vi "PC_Main.vi"() -> ()   [LabVIEW 2018]
uses:
  Type Defs/measurement states.ctl
  Type Defs/Processing Settings 1.ctl
  <vilib>/Analysis/baseanly.llb/Mean (DBL).vi
  <vilib>/WebDAVClient/Simple Get Buffer.vi
  <vilib>/WebDAVClient/NI_WebDAV.lvlib
  Alignment Mode Window.vi
  Update Settings.vi
  <vilib>/Analysis/NI_AALBase.lvlib
panel:
  in  "Settings":bool
  in  "Alignment":bool
  in  "Start Button":bool
  in  "STOP":bool
  in  "Choose Correction":bool caption="Calculated              Calibration\nCorrection                Correction"
  in  "Sensor Select":bool
  in  "Repeat\nMeasurement":bool
  out "Meas. Complete":bool
  out "Waiting For Data":bool
  out "Detection Failure":bool=TRUE
  out "Peaks":cluster{"Locations":dbl[], "Amplitudes":dbl[]}[](graph)
  out "Mean Thickness (µm)":dbl format="%.2g"
  out "Thickness Array":dbl[](array[numeric]) format="%.2g"
  in  "N Tests":i32
  in  "alignment off":bool
  out "Thickness (µm)":dbl format="%.2g"
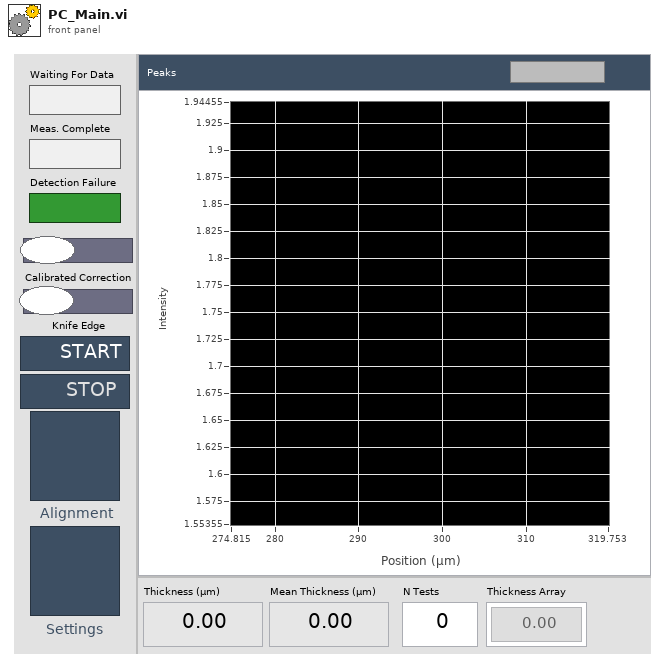
[diagram p1: front panel]
types:
  T1 = typedef "Processing Settings 1.ctl" = cluster{"Edlen\nSettings":cluster{"P_atm":i32, "T (deg C)":i32, "PP h20":dbl}, "Processing\nSettings":cluster{"Subset Length":i32, "Peak Width":i32, "Filter Width":i32, "Threshold (V)":dbl}}
  T2 = typedef "measurement states.ctl" = enum16{"reset alignment mode", "sensor select", "start measurement", "alignment", "configure", "idle", "wait for data", "load data", "process data", "exit", "find peaks"}
  T3 = cluster{"Moving Averaged Array":dbl[], "Moving Averaged Array":dbl[]}
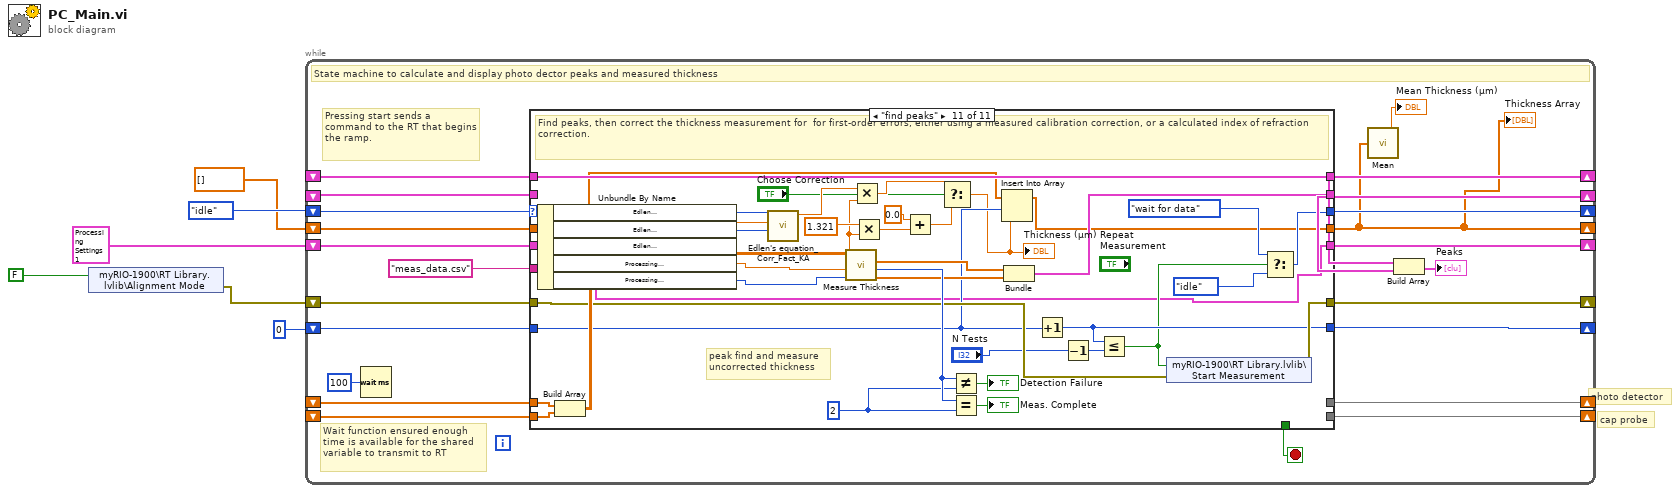
[diagram p0: block diagram]
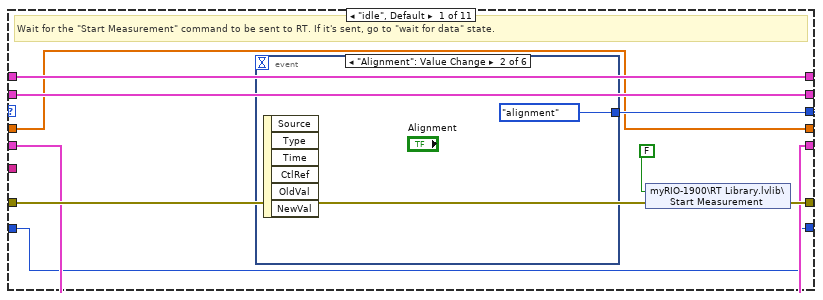
[diagram p2: hidden frame]
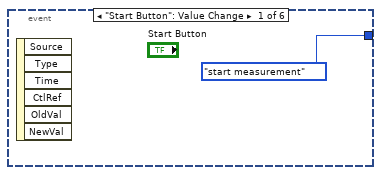
[diagram p3: hidden frame]
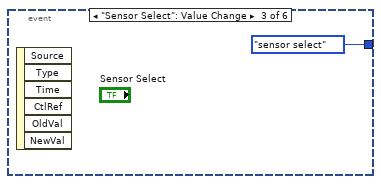
[diagram p4: hidden frame]
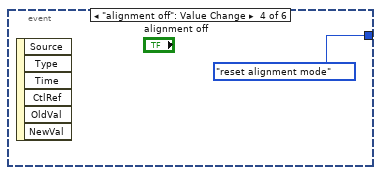
[diagram p5: hidden frame]
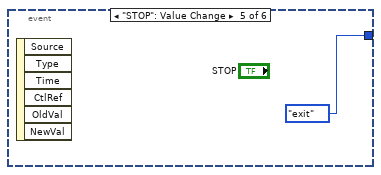
[diagram p6: hidden frame]
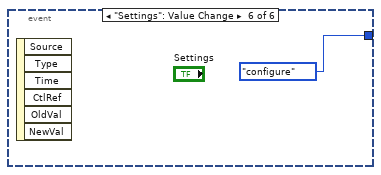
[diagram p7: hidden frame]
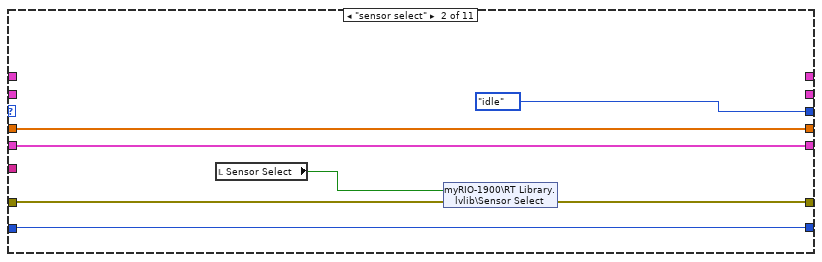
[diagram p8: hidden frame]
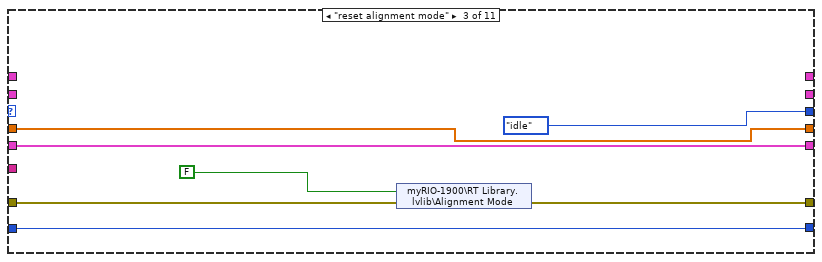
[diagram p9: hidden frame]
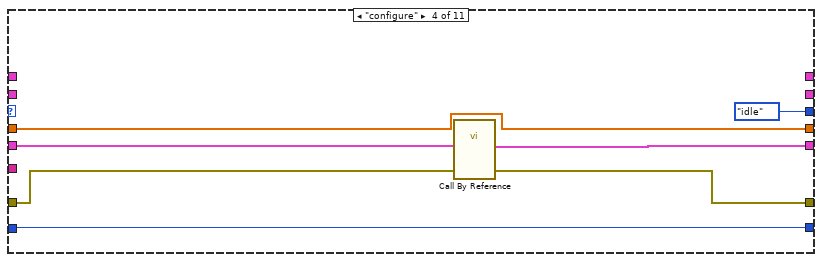
[diagram p10: hidden frame]
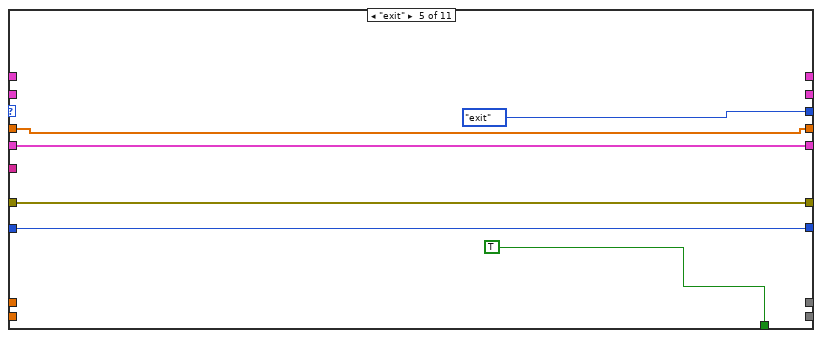
[diagram p11: hidden frame]
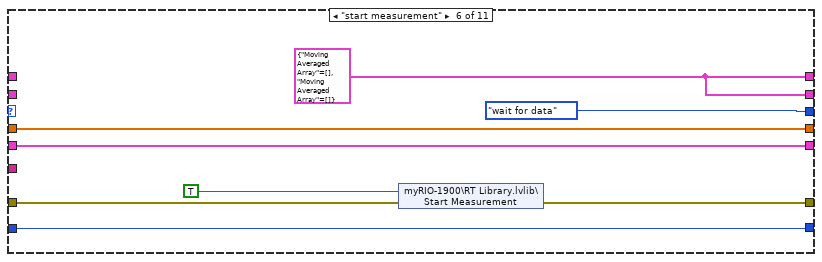
[diagram p12: hidden frame]
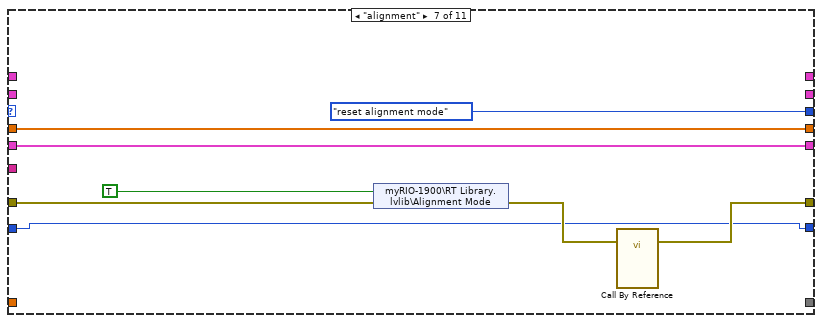
[diagram p13: hidden frame]
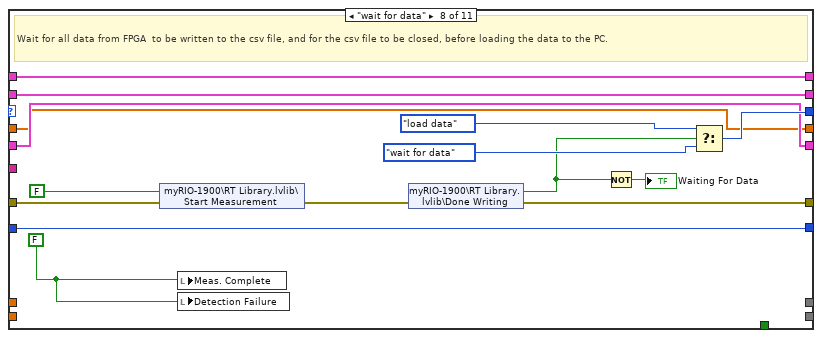
[diagram p14: hidden frame]
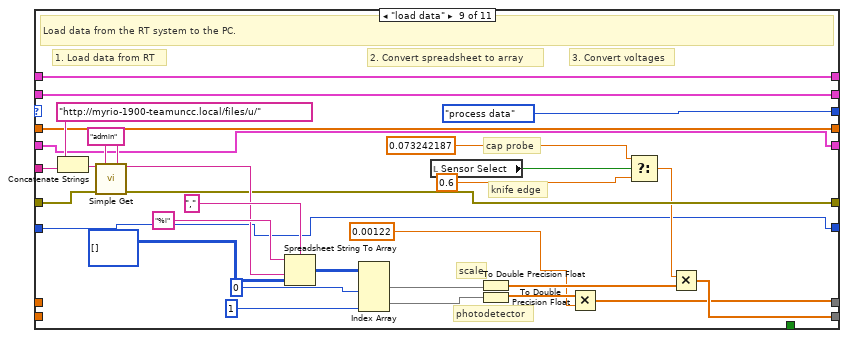
[diagram p15: hidden frame]
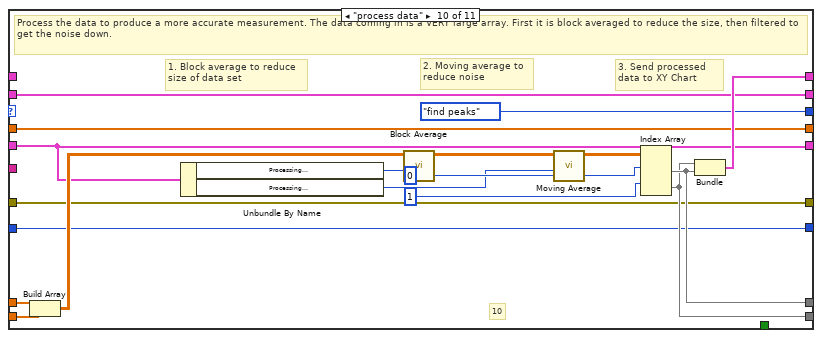
[diagram p16: hidden frame]
diagram:
  # "photo detector"
  # "cap probe"
  n1 = shared-variable "myRIO-1900\\RT Library.lvlib\\Alignment Mode"(FALSE) -> (error out=w4:errorcluster)  [unwired: 1 in]
  n2 = while {
    shift-right: [w28] -> _
    shift-left: measurement_states."idle" ("Enum") -> [w29]
    shift-right: [w27] -> _
    shift-left: w4 -> [w15]
    shift-right: [w25] -> _
    shift-left: _ -> [w24]
    shift-right: [w26] -> _
    shift-left: _ -> [w23]
    shift-right: [w18] -> _
    shift-left: _ -> [w17]
    shift-right: [w19] -> _
    shift-left: _ -> [w16]
    shift-right: [w10] -> _
    shift-left: dbl[] [] -> [w13]
    shift-right: [w11] -> _
    shift-left: 0 -> [w12]
    shift-right: [w7] -> _
    shift-left: T1 {"Edlen\nSettings"={"P_atm"=100, "T (deg C)"=50, "PP h20"=100.0}, "Processing\nSettings"={"Subset Length"=1, "Peak Width"=50, "Filter Width"=100, "Threshold (V)"=0.8}} ("Processing\nSettings") -> [w8]
    stop <- w14 stop-if-true
    # "Wait function ensured enough time is available for the shared variable to transmit to RT"
    # "Pressing start sends a command to the RT that begins the ramp."
    # "State machine to calculate and display photo dector peaks and measured thickness"
    n3 = Wait (ms)(milliseconds to wait=u32 100) -> ()  [unwired: 1 out]
    n4 = case shown="\"find peaks\"" w29 {
      tunnel: [w36 measurement_states."idle" ("Enum") measurement_states."idle" ("Enum") measurement_states."idle" ("Enum") measurement_states."exit" ("Enum") measurement_states."wait for data" ("Enum") measurement_states."reset alignment mode" ("Enum") w101 measurement_states."process data" measurement_states."find peaks" w175] -> w28
      tunnel: [w33 w50 w56 w63 w68 w79 w83 w97 w120 w141 w173] -> w27
      tunnel: [_ _ _ _ _ _ _ _ w117 w142 _] -> w25
      tunnel: [_ _ _ _ _ _ _ _ w114 w143 _] -> w26
      tunnel: w24 -> [_ _ _ _ _ _ _ _ _ w148 w187]
      tunnel: w23 -> [_ _ _ _ _ _ _ _ _ w149 w188]
      tunnel: "meas_data.csv" ("File Name") -> [_ _ _ _ _ _ _ _ w118 _ _]
      tunnel: w15 -> [w34 w51 w57 w64 w68 w78 w87 w92 w113 w141 w174]
      tunnel: [w38 _ _ _ _ w74 _ w94 w112 w140 w178] -> w19
      tunnel: [w37 _ _ _ _ w74 _ w95 w111 w139 w179] -> w18
      tunnel: w17 -> [w37 _ _ _ _ _ _ w95 w111 w139 _]
      tunnel: w16 -> [w38 _ _ _ _ _ _ w94 w112 _ w178]
      tunnel: [_ _ _ _ TRUE _ _ _ _ _ _] -> w14
      tunnel: w8 -> [w32 w47 w54 w59 w69 w75 w82 w90 w106 w135 w158]
      tunnel: [w32 w47 w54 w60 w69 w75 w82 w90 w106 w135 w158] -> w7
      tunnel: [w31 w46 w53 w62 w67 w73 w81 w89 w105 w134 w172] -> w10
      tunnel: w13 -> [w31 w46 w53 w62 w67 w73 w81 w89 w105 w134 w171]
      tunnel: w12 -> [w30 w45 w52 w61 w66 w72 w80 w88 w104 w133 w170]
      tunnel: [w30 w45 w52 w61 w66 w72 w80 w88 w104 w133 w169] -> w11
      frame "idle", Default {
        # "Wait for the \"Start Measurement\" command to be sent to RT. If it's sent, go to \"wait for data\" state."
        n5 = event shown="[1] \"Alignment\": Value Change" {
          selector: _ -> [_ _ _ _ _ _]
          dyn-events: _ -> [_ _ _ _ _ _]
          timeout: _ -> [_ _ _ _ _ _]
          tunnel: [measurement_states."start measurement" ("Enum") measurement_states."alignment" ("Enum") measurement_states."sensor select" ("Enum") measurement_states."reset alignment mode" ("Enum") measurement_states."exit" ("Enum") measurement_states."configure" ("Enum")] -> w36
          event "Start Button": Value Change {
            n6 = event-data() -> ()  [unwired: 1 in, 6 out]
          }
          event "Alignment": Value Change {
            n7 = event-data() -> ()  [unwired: 1 in, 6 out]
          }
          event "Sensor Select": Value Change {
            n8 = event-data() -> ()  [unwired: 1 in, 6 out]
          }
          event "alignment off": Value Change {
            n9 = event-data() -> ()  [unwired: 1 in, 6 out]
          }
          event "STOP": Value Change {
            n10 = event-data() -> ()  [unwired: 1 in, 6 out]
          }
          event "Settings": Value Change {
            n11 = event-data() -> ()  [unwired: 1 in, 6 out]
          }
        }
        n12 = shared-variable "myRIO-1900\\RT Library.lvlib\\Start Measurement"(FALSE, error in=w34) -> (error out=w33:errorcluster)
      }
      frame "sensor select" {
        n13 = local read "Sensor Select"() -> (w49:bool)
        n14 = shared-variable "myRIO-1900\\RT Library.lvlib\\Sensor Select"(w49, error in=w51) -> (error out=w50:errorcluster)
      }
      frame "reset alignment mode" {
        n15 = shared-variable "myRIO-1900\\RT Library.lvlib\\Alignment Mode"(FALSE, error in=w57) -> (error out=w56:errorcluster)
      }
      frame "configure" {
        n16 = call-by-ref "?"("error in (no error)"=w64, "Processing\nSettings 2"=w59) -> ("error out"=w63:errorcluster, "Processing\nSettings Out"=w60:T1)  [unwired: 10 in, 2 out]
      }
      frame "exit" {
      }
      frame "start measurement" {
        w74 = T3 {"Moving Averaged Array"=[], "Moving Averaged Array"=[]}
        n17 = shared-variable "myRIO-1900\\RT Library.lvlib\\Start Measurement"(TRUE, error in=w78) -> (error out=w79:errorcluster)
      }
      frame "alignment" {
        n18 = shared-variable "myRIO-1900\\RT Library.lvlib\\Alignment Mode"(TRUE, error in=w87) -> (error out=w84:errorcluster)
        n19 = call-by-ref "?"(error in=w84) -> (error out=w83:errorcluster)  [unwired: 13 in, 1 out]
      }
      frame "wait for data" {
        w96 = FALSE
        # "Wait for all data from FPGA  to be written to the csv file, and for the csv file to be closed, before loading the data to the PC."
        n20 = shared-variable "myRIO-1900\\RT Library.lvlib\\Start Measurement"(FALSE, error in=w92) -> (error out=w91:errorcluster)
        n21 = local write "Meas. Complete"(w96) -> ()
        n22 = local write "Detection Failure"(w96) -> ()
        n23 = shared-variable "myRIO-1900\\RT Library.lvlib\\Done Writing"(error in=w91) -> (w99:bool, error out=w97:errorcluster)
        n24 = Not(x=w99) -> (.not. x?=→"Waiting For Data":bool)
        n25 = Select(t=measurement_states."load data", s=w99, f=measurement_states."wait for data") -> (s? t:f=w101:T2)
      }
      frame "load data" {
        w132 = "admin" ("username")
        # "knife edge"
        # "cap probe"
        # "3. Convert voltages"
        # "2. Convert spreadsheet to array"
        # "1. Load data from RT"
        # "photodetector"
        # "scale"
        # "Load data from the RT system to the PC."
        n26 = Concatenate Strings("http://myrio-1900-teamuncc.local/files/u/" ("address"), w118) -> (w125:string)
        n27 = call-poly <vilib>:"Simple Get.vi"("remote file uri"=w125, "username"=w132, "password"=w132, "error in (no error)"=w113) -> ("data"=w128:string, "error out"=w120:errorcluster)  [unwired: 10 in]
        n28 = Spreadsheet String To Array(delimiter (Tab)=",", format string="%i", spreadsheet string=w128, array type (2D Dbl)=i32[][] []) -> (array=w127:i32[][])
        n29 = Index Array(array=w127, index (col) #1=0 ("disabled index (col)"), index (col) #2=1 ("index (col)")) -> (element #1=w123:i32[], element #2=w122:i32[])  [unwired: 2 in]
        n30 = local read "Sensor Select"() -> (w108:bool)
        n31 = To Double Precision Float(number=w123) -> (double precision float=w121:dbl[])
        n32 = To Double Precision Float(number=w122) -> (double precision float=w116:dbl[])
        n33 = Multiply(x=w116, y=0.00122 ("x")) -> (x*y=w114:dbl[])
        n34 = Select(t=0.073242187 ("x"), s=w108, f=0.6 ("x")) -> (s? t:f=w107:dbl)
        n35 = Multiply(x=w107, y=w121) -> (x*y=w117:dbl[])
      }
      frame "process data" {
        # "3. Send processed data to XY Chart"
        # "10"
        # "2. Moving average to reduce noise"
        # "1. Block average to reduce\nsize of data set"
        # "Process the data to produce a more accurate measurement. The data coming in is a VERY large array. First it is block averaged to reduce the size, then filtered to get the noise down."
        n36 = Build Array(w149, w148) -> (w147:dbl[][])
        n37 = Unbundle By Name(w135) -> ("Processing\nSettings.Subset Length"=w137:i32, "Processing\nSettings.Filter Width"=w136:i32)
        n38 = call "Block Average.vi"("Subset Length"=w137, "Input Array"=w147) -> ("Block Averaged Array"=w150:dbl[][])  [unwired: 9 in]
        n39 = call "Moving Average.vi"("Filter Width"=w136, "Input Array"=w150) -> ("Moving Averaged Array"=w146:dbl[][])  [unwired: 9 in]
        n40 = Index Array(array=w146, index (row) #1=0 ("disabled index (col)"), index (row) #2=1 ("index (col)")) -> (element #1=w143:dbl[], element #2=w142:dbl[])  [unwired: 2 in]
        n41 = Bundle("Moving Averaged Array"=w142, "Moving Averaged Array"=w143) -> (w140:T3)  [unwired: 1 in]
      }
      frame "find peaks" {
        w183 = 2
        # "peak find and measure\nuncorrected thickness"
        # "Find peaks, then correct the thickness measurement for  for first-order errors, either using a measured calibration correction, or a calculated index of refraction correction."
        n42 = Unbundle By Name(w158) -> ("Edlen\nSettings.T (deg C)"=w157:i32, "Edlen\nSettings.PP h20"=w156:dbl, "Edlen\nSettings.P_atm"=w155:i32, "Processing\nSettings.Threshold (V)"=w154:dbl, "Processing\nSettings.Peak Width"=w153:i32)
        n43 = Build Array(w188, w187) -> (w186:dbl[][])
        n44 = call "Edlen's equation_Corr_Fact_KA.vi"("pressure (Pa)"=w155, "f, partial pressure of water (Pa)"=w156, "Temperature (degC)"=w157) -> ("Correction Factor"=w159:dbl)  [unwired: 8 in]
        n45 = call "Measure Thickness.vi"("peak detector width"=w153, "threshold"=w154, "Input Array"=w186) -> ("Amplitudes"=w180:dbl[], "peaks found"=w184:i32, "Locations"=w181:dbl[], "uncorrected thickness"=w163:dbl)  [unwired: 5 in]
        n46 = Multiply(x=w159, y=w163) -> (x*y=w165:dbl)
        n47 = Multiply(x=1.321 ("f"), y=w163) -> (x*y=w162:dbl)
        n48 = Add(x=0.0, y=w162) -> (x+y=w160:dbl)
        n49 = Select(t=w165, s="Choose Correction", f=w160) -> (s? t:f=w166:dbl)
        "Thickness (µm)" <- w166
        n50 = Not Equal?(x=w184, y=w183) -> (x != y?=→"Detection Failure":bool)
        n51 = Equal?(x=w184, y=w183) -> (x = y?=→"Meas. Complete":bool)
        n52 = Insert Into Array(array=w171, index=w170, new element=w166) -> (w172:dbl[])
        n53 = Bundle("Locations"=w181, "Amplitudes"=w180) -> (w179:cluster{"Locations":dbl[], "Amplitudes":dbl[]})  [unwired: 1 in]
        n54 = Increment(x=w170) -> (x+1=w169:i32)
        n55 = Decrement(x="N Tests") -> (x-1=w167:i32)
        n56 = Less Or Equal?(x=w169, y=w167) -> (x <= y?=w168:bool)
        n57 = shared-variable "myRIO-1900\\RT Library.lvlib\\Start Measurement"(w168, error in=w174) -> (error out=w173:errorcluster)
        n58 = Select(t=measurement_states."wait for data" ("Enum"), s=w168, f=measurement_states."idle" ("Enum")) -> (s? t:f=w175:T2)
      }
    }
    "Thickness Array" <- w10
    n59 = call-poly <vilib>:"Mean.vi"("X"=w10) -> ("mean"=→"Mean Thickness (µm)":dbl)  [unwired: 1 out]
    n60 = Build Array(w19, w18) -> (→"Peaks":cluster{"Locations":dbl[], "Amplitudes":dbl[]}[])
  }
